vi "GetDescription.vi"(0 "reference in":refnum<class "CondimentDecorator.lvclass">, 5 "error in (no error)":errorcluster) -> (14 "reference out":refnum<class "CondimentDecorator.lvclass">, 16 "Description":string, 19 "error out":errorcluster)   [LabVIEW 2020, in "CondimentDecorator.lvclass"]
uses:
  CondimentDecorator.lvclass
  Beverage_class/Beverage.lvclass
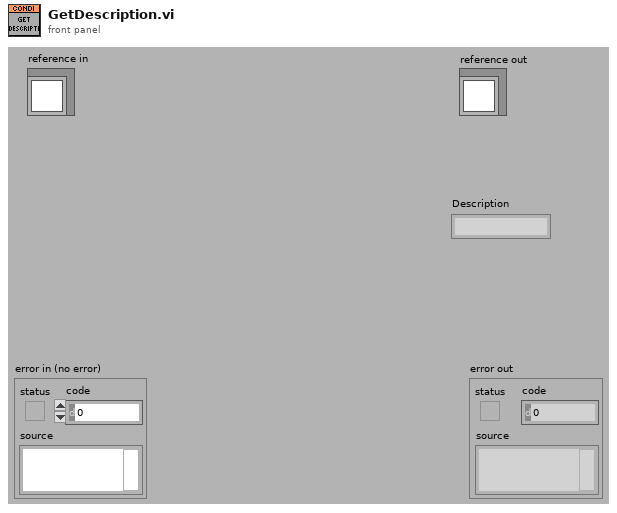
[diagram p1: front panel]
types:
  T1 = typedef "CondimentDecorator.lvclass/ObjectAttributes.ctl" = cluster{"BeverageRef":refnum<class "Beverage.lvclass">, "CondimentName":string}
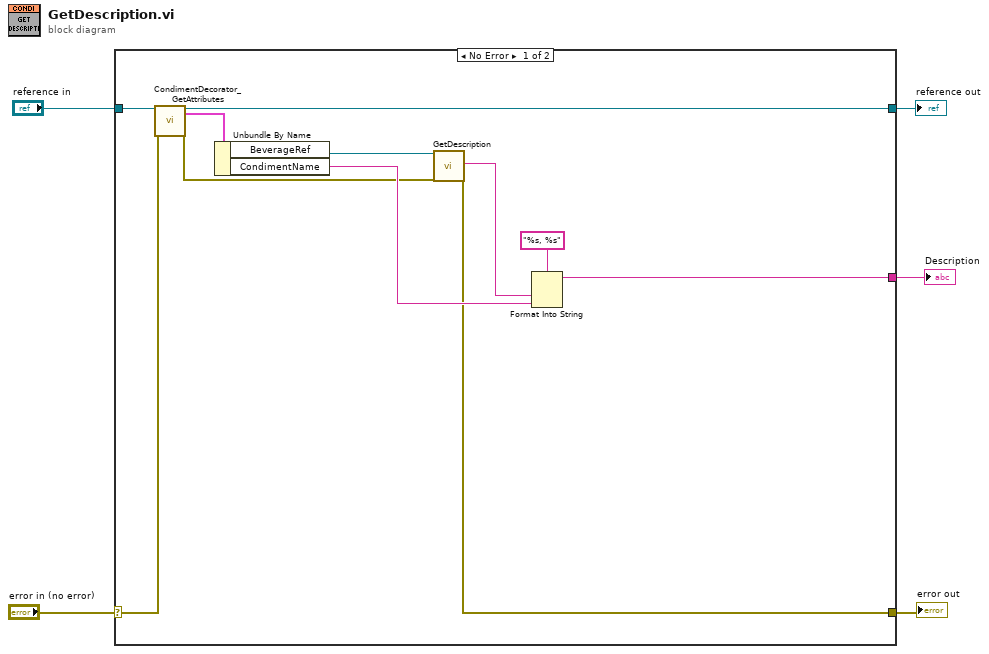
[diagram p0: block diagram]
diagram:
  n1 = case shown="No Error" "error in (no error)" {
    selector: "error in (no error)" -> [w16 w18]
    tunnel: [w8 w18] -> w4
    tunnel: [w13 w17] -> w2
    tunnel: "reference in" -> [w14 w17]
    tunnel: [w7 _] -> w1
    frame No Error {
      n2 = call "CondimentDecorator_GetAttributes.vi"("reference in"=w14, "error in (no error)"=w16) -> ("reference out"=w13:refnum<class "CondimentDecorator.lvclass">, "Data"=w15:T1, "error out"=w9:errorcluster)  [unwired: 14 in, 1 out]
      n3 = Unbundle By Name(w15) -> ("BeverageRef"=w11:refnum<class "Beverage.lvclass">, "CondimentName"=w10:string)
      n4 = call-dynamic "GetDescription.vi"("reference in"=w11, "error in (no error)"=w9) -> ("Description"=w6:string, "error out"=w8:errorcluster)  [unwired: 15 in, 1 out]
      n5 = Format Into String(format string="%s, %s", w6, w10) -> (resulting string=w7:string)  [unwired: 2 in, 1 out]
    }
    frame Error {
    }
  }
  "error out" <- w4
  "reference out" <- w2
  "Description" <- w1
